vi "Interface.vi"(2 "error in":errorcluster, 3 "Values":T1, 4 "Arduino Resource":T3={"VISA resource"="", "Board Type"=enum."Uno", "Connection Type"=enum."USB / Serial", "Bytes Per Packet (15)"=15}) -> (0 "error out":errorcluster, 1 "Arduino Resource":T3={"VISA resource"="", "Board Type"=enum."Uno", "Connection Type"=enum."USB / Serial", "Bytes Per Packet (15)"=15})   [LabVIEW 2013]
uses:
  <vilib>/LabVIEW Interface for Arduino/Type Defs/Arduino Resource.ctl
  <vilib>/LabVIEW Interface for Arduino/Type Defs/Board Type.ctl
  <vilib>/LabVIEW Interface for Arduino/Type Defs/Pin Mode.ctl
  <vilib>/LabVIEW Interface for Arduino/LabVIEW Interface for Arduino.lvlib
panel:
  in  "Modes":T2[](array[typedef])
  in  "Pins":u8[](array[numeric])=[8, 9, 10, 11]
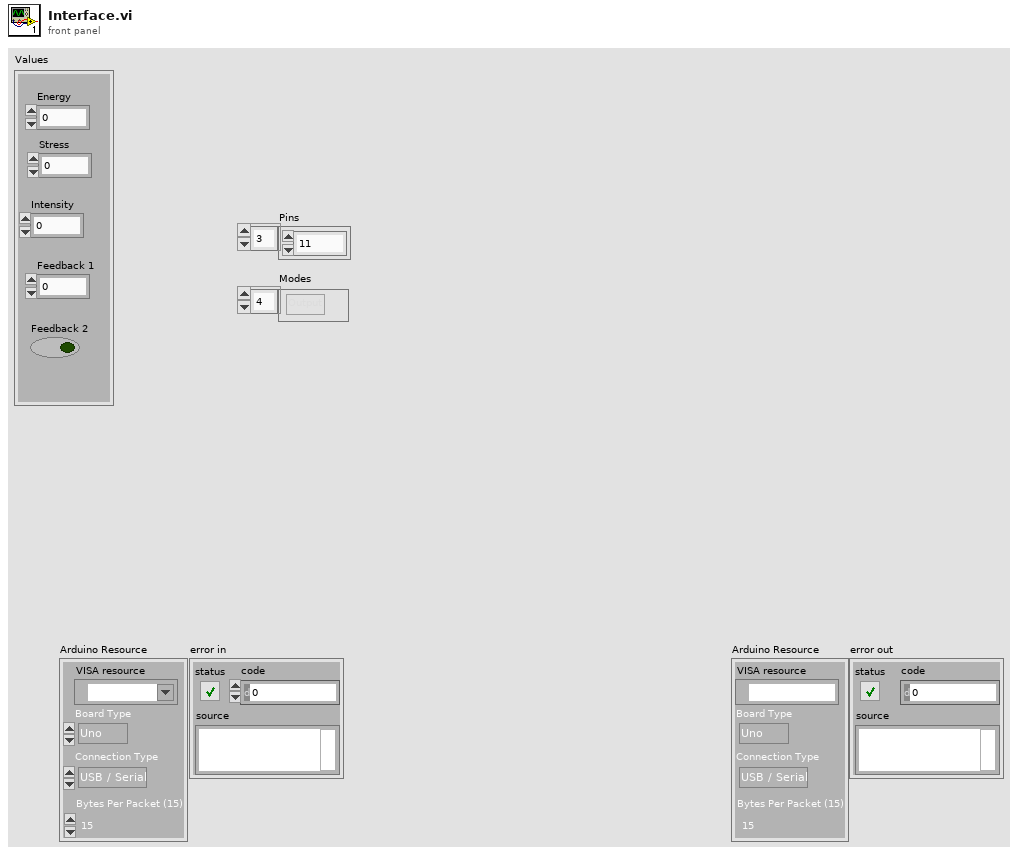
[diagram p1: front panel]
types:
  T1 = cluster{"Energy":dbl, "Stress":dbl, "Intensity":dbl, "Feedback 1":dbl, "Feedback 2":bool}
  T2 = typedef "LabVIEW Interface for Arduino.lvlib/Pin Mode.ctl" = enum8{"Input", "Output"}
  T3 = typedef "LabVIEW Interface for Arduino.lvlib/Arduino Resource.ctl" = cluster{"VISA resource":refnum<visa-resource-name>, "Board Type":T4, "Connection Type":enum8{"USB / Serial"}, "Bytes Per Packet (15)":u8}
  T4 = typedef "LabVIEW Interface for Arduino.lvlib/Board Type.ctl" = enum16{"Uno", "Dimuelanove w/Atmega 328", "Mega 2560"}
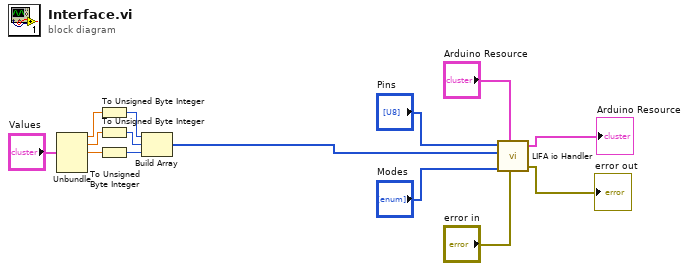
[diagram p0: block diagram]
diagram:
  n1 = Unbundle("Values") -> ("Energy"=w5:dbl, "Stress"=w4:dbl, "Intensity"=w3:dbl)  [unwired: 2 out]
  n2 = To Unsigned Byte Integer(number=w5) -> (unsigned 8bit integer=w10:u8)
  n3 = To Unsigned Byte Integer(number=w4) -> (unsigned 8bit integer=w9:u8)
  n4 = To Unsigned Byte Integer(number=w3) -> (unsigned 8bit integer=w8:u8)
  n5 = Build Array(w10, w9, w8) -> (w7:u8[])
  n6 = call "LIFA io Handler.vi"("Pins"="Pins", "Arduino Resource"="Arduino Resource", "Values"=w7, "error in"="error in", "Modes"="Modes") -> ("Arduino Resource"=→"Arduino Resource":T3, "error out"=→"error out":errorcluster)  [unwired: 2 in]
